vi "Bitfile SLSC Interfaces.vi"(11 "SLSC CD Version":T1) -> (2 "IP Types":T2[](array[typedef]), 3 "IP Interface":variant[](array[variant]))   [LabVIEW 2014, in "SLSC configuration System Explorer.lvlib"]
uses:
  SLSC configuration System Explorer.lvlib
  Type Defs/Register Types.ctl
  Type Defs/SLSC Custom Device Version.ctl
  Example/SPI API Test/FPGA/SLSC FPGA Inputs.ctl
  <userlib>/_NI SPI IP/FPGA/Controllers/Public/Transfer Settings.ctl
  Example/SPI API Test/FPGA/SLSC # of racks.ctl
  Example/SPI API Test/FPGA/SLSC FIFO name.ctl
  Example/SPI API Test/FPGA/SLSC UEGO Calibration.ctl
  <userlib>/_NI SPI IP/FPGA/Controllers/NI SPI IP FPGA.lvlib
  Example/SPI API Test/FPGA/SLSC FPGA Toolkit.lvlib
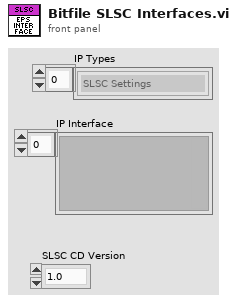
[diagram p1: front panel]
types:
  T1 = typedef "SLSC configuration System Explorer.lvlib/SLSC Custom Device Version.ctl" = enum8{"1.0"}
  T2 = typedef "SLSC configuration System Explorer.lvlib/Register Types.ctl" = enum16{"SLSC Settings", "# of Racks", "SPI FIFO Name", "UEGO Calibration"}
  T3 = typedef "SLSC FPGA Toolkit.lvlib/SLSC FPGA Inputs.ctl" = cluster{"SPI PHY Settings":T4, "Sample Rate (S/s)":u32}
  T4 = typedef "NI SPI IP FPGA.lvlib/Transfer Settings.ctl" = cluster{"Divide Value":u8, "Transfer Length (bits)":u8, "CS Asserted Polarity":bool, "Clock Polarity (CPOL)":bool, "Clock Phase (CPHA)":bool, "Lengthen MISO Setup":bool, "Direction Change Bit":u8, "MOSI Starts as Output":bool, "Tristatable MOSI":bool}
  T5 = typedef "SLSC FPGA Toolkit.lvlib/SLSC # of racks.ctl" = cluster{"# of Racks":bool}
  T6 = typedef "SLSC FPGA Toolkit.lvlib/SLSC FIFO name.ctl" = cluster{"FIFO Name":bool}
  T7 = typedef "SLSC FPGA Toolkit.lvlib/SLSC UEGO Calibration.ctl" = cluster{"Rack #":u8, "CS Bit Value/Slot #":u8, "Calibration Ticks":u16, "HW Settling Ticks":u16}
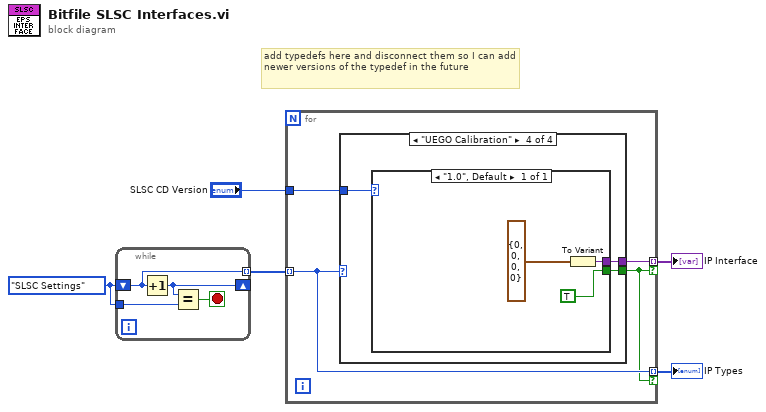
[diagram p0: block diagram]
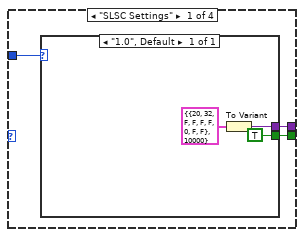
[diagram p2: hidden frame]
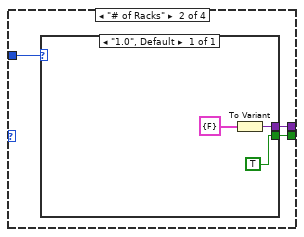
[diagram p3: hidden frame]
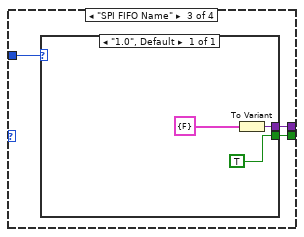
[diagram p4: hidden frame]
diagram:
  w4 = Register_Types."SLSC Settings" ("Register Types")
  # "add typedefs here and disconnect them so I can add newer versions of the typedef in the future"
  n1 = while {
    shift-right: [w7] -> _
    shift-left: w4 -> [w9]
    tunnel: [w9] -> w3 mode=indexing
    tunnel: w4 -> [w6]
    stop <- w8 stop-if-true
    n2 = Increment(x=w9) -> (x+1=w7:T2)
    n3 = Equal?(x=w7, y=w6) -> (x = y?=w8:bool)
  }
  n4 = for {
    tunnel: w3 -> [w11] mode=indexing
    tunnel: "SLSC CD Version" -> [w13]
    tunnel: [w12] -> w2 mode=indexing if=w10
    tunnel: [w11] -> w1 mode=indexing if=w10
    n5 = case shown="\"UEGO Calibration\"" w11 {
      tunnel: w13 -> [w16 w22 w28 w34]
      tunnel: [w15 w21 w27 w33] -> w12
      tunnel: [w14 w20 w26 w32] -> w10
      frame "SLSC Settings" {
        n6 = case shown="\"1.0\", Default" w16 {
          tunnel: [w17] -> w15
          tunnel: [TRUE ("done")] -> w14
          frame "1.0", Default {
            n7 = To Variant(anything=T3 {"SPI PHY Settings"={"Divide Value"=20, "Transfer Length (bits)"=32, "CS Asserted Polarity"=FALSE, "Clock Polarity (CPOL)"=FALSE, "Clock Phase (CPHA)"=FALSE, "Lengthen MISO Setup"=FALSE, "Direction Change Bit"=0, "MOSI Starts as Output"=FALSE, "Tristatable MOSI"=FALSE}, "Sample Rate (S/s)"=10000} ("settings with acceleration")) -> (Variant=w17:variant)
          }
        }
      }
      frame "# of Racks" {
        n8 = case shown="\"1.0\", Default" w22 {
          tunnel: [w25] -> w21
          tunnel: [TRUE ("done")] -> w20
          frame "1.0", Default {
            n9 = To Variant(anything=T5 {"# of Racks"=FALSE} ("APU Shared Settings")) -> (Variant=w25:variant)
          }
        }
      }
      frame "SPI FIFO Name" {
        n10 = case shown="\"1.0\", Default" w28 {
          tunnel: [w31] -> w27
          tunnel: [TRUE ("done")] -> w26
          frame "1.0", Default {
            n11 = To Variant(anything=T6 {"FIFO Name"=FALSE}) -> (Variant=w31:variant)
          }
        }
      }
      frame "UEGO Calibration" {
        n12 = case shown="\"1.0\", Default" w34 {
          tunnel: [w37] -> w33
          tunnel: [TRUE ("done")] -> w32
          frame "1.0", Default {
            n13 = To Variant(anything=T7 {"Rack #"=0, "CS Bit Value/Slot #"=0, "Calibration Ticks"=0, "HW Settling Ticks"=0}) -> (Variant=w37:variant)
          }
        }
      }
    }
  }
  "IP Types" <- w1
  "IP Interface" <- w2
